vi "ReadArray.vi"(1 "reference":refnum<vi>) -> (0 "Array":T6)   [LabVIEW 2013]
uses:
  <vilib>/Utility/miscctls.llb/LVBoundsTypeDef.ctl
  <vilib>/Utility/miscctls.llb/LVPositionTypeDef.ctl
  <vilib>/Utility/miscctls.llb/LVRectTypeDef.ctl
  <vilib>/Utility/miscctls.llb/LVDataSocketStatusTypeDef.ctl
  <vilib>/Utility/miscctls.llb/LVKeyNavTypeDef.ctl
panel:
  out "error out 74":errorcluster
  out "error out 73":errorcluster
  out "error out 72":errorcluster
  out "error out 71":errorcluster
  out "error out 70":errorcluster
  out "error out 69":errorcluster
  out "error out 68":errorcluster
  out "error out 67":errorcluster
  out "error out 66":errorcluster
  out "error out 65":errorcluster
  out "error out 64":errorcluster
  out "error out 63":errorcluster
  out "error out 62":errorcluster
  out "error out 61":errorcluster
  out "error out 60":errorcluster
  out "error out 59":errorcluster
  out "error out 58":errorcluster
  out "error out 57":errorcluster
  out "error out 56":errorcluster
  out "error out 55":errorcluster
  out "error out 54":errorcluster
  out "error out 53":errorcluster
  out "error out 52":errorcluster
  out "error out 51":errorcluster
  out "error out 50":errorcluster
  out "error out 49":errorcluster
  out "error out 48":errorcluster
  out "error out 47":errorcluster
  out "error out 46":errorcluster
  out "error out 45":errorcluster
  out "error out 44":errorcluster
  out "error out 43":errorcluster
  out "error out 42":errorcluster
  out "error out 41":errorcluster
  out "error out 40":errorcluster
  out "error out 39":errorcluster
  out "error out 38":errorcluster
  out "error out 37":errorcluster
  out "error out 36":errorcluster
  out "error out 35":errorcluster
  out "error out 34":errorcluster
  out "error out 33":errorcluster
  out "error out 32":errorcluster
  out "error out 31":errorcluster
  out "error out 30":errorcluster
  out "error out 29":errorcluster
  out "error out 28":errorcluster
  out "error out 27":errorcluster
  out "error out 26":errorcluster
  out "error out 25":errorcluster
  out "error out 24":errorcluster
  out "error out 23":errorcluster
  out "error out 22":errorcluster
  out "error out 21":errorcluster
  out "error out 20":errorcluster
  out "error out 19":errorcluster
  out "error out 18":errorcluster
  out "error out 17":errorcluster
  out "error out 16":errorcluster
  out "error out 15":errorcluster
  out "error out 14":errorcluster
  out "error out 13":errorcluster
  out "error out 12":errorcluster
  out "error out 11":errorcluster
  out "error out 10":errorcluster
  out "error out 9":errorcluster
  out "error out 8":errorcluster
  out "error out 7":errorcluster
  out "error out 6":errorcluster
  out "error out 5":errorcluster
  out "error out 4":errorcluster
  out "error out 3":errorcluster
  out "error out 2":errorcluster
  out "error out":errorcluster
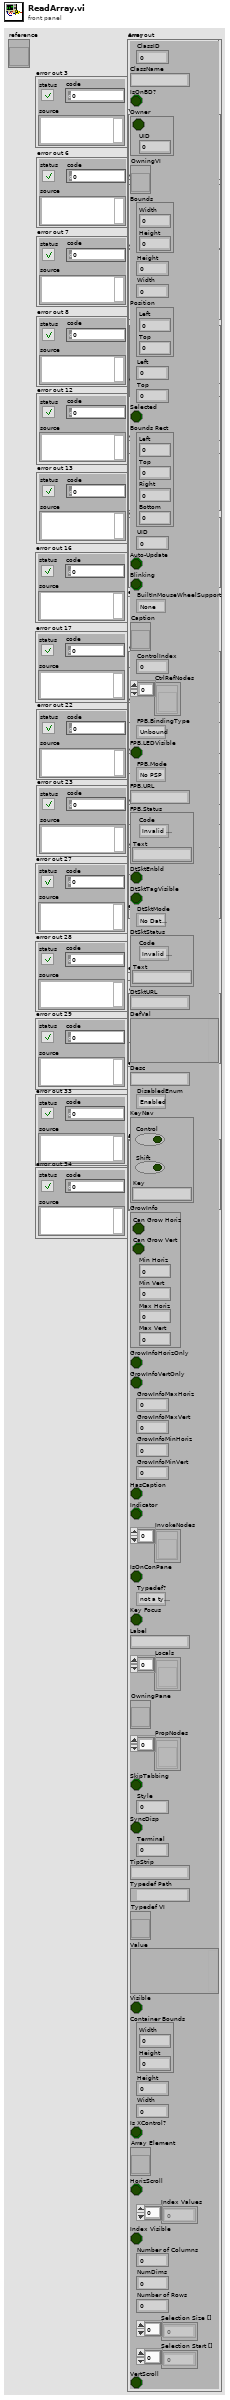
[diagram p1: front panel]
types:
  T1 = typedef "LVBoundsTypeDef.ctl" = cluster{"Width":u32, "Height":u32}
  T2 = typedef "LVPositionTypeDef.ctl" = cluster{"Left":i32, "Top":i32}
  T3 = typedef "LVRectTypeDef.ctl" = cluster{"Left":i16, "Top":i16, "Right":i16, "Bottom":i16}
  T4 = typedef "LVDataSocketStatusTypeDef.ctl" = cluster{"Code":enum32{"Invalid Status", "Unconnected", "Active", "Idle", "Error", "Connecting"}, "Text":string}
  T5 = typedef "LVKeyNavTypeDef.ctl" = cluster{"Control":bool, "Shift":bool, "Key":string}
  T6 = cluster{"ClassID":u32, "ClassName":string, "IsOnBD?":bool, "Owner":cluster{bool, "UID":i32}, "OwningVI":refnum<vi>, "Bounds":T1, "Height":u32, "Width":u32, "Position":T2, "Left":i32, "Top":i32, "Selected":bool, "Bounds Rect":T3, "UID":i32, "Auto-Update":bool, "Blinking":bool, "BuiltInMouseWheelSupport":enum16{"None", "On Hover", "On Key Focus", "On Hover or Key Focus"}, "Caption":refnum<vi>, "ControlIndex":i32, "CtrlRefNodes":refnum<vi>[], "FPB.BindingType":enum32{"Unbound", "Bound To PSP URL", "Bound To Variable Shortcut"}, "FPB.LEDVisible":bool, "FPB.Mode":enum32{"No PSP", "Read", "Write", "Write & Read"}, "FPB.URL":string, "FPB.Status":T4, "DtSktEnbld":bool, "DtSktTagVisible":bool, "DtSktMode":enum32{"No DataSocket", "Publish", "Subscribe", "Publish & Subscribe"}, "DtSktStatus":T4, "DtSktURL":string, "DefVal":variant, "Desc":string, "DisabledEnum":enum8{"Enabled", "Disabled", "Disabled and Grayed Out"}, "KeyNav":T5, "GrowInfo":cluster{"Can Grow Horiz":bool, "Can Grow Vert":bool, "Min Horiz":i16, "Min Vert":i16, "Max Horiz":i16, "Max Vert":i16}, "GrowInfoHorizOnly":bool, "GrowInfoVertOnly":bool, "GrowInfoMaxHoriz":i16, "GrowInfoMaxVert":i16, "GrowInfoMinHoriz":i16, "GrowInfoMinVert":i16, "HasCaption":bool, "Indicator":bool, "InvokeNodes":refnum<vi>[], "IsOnConPane":bool, "Typedef?":enum32{"not a typedef", "typedef", "strict typedef", "class private data"}, "Key Focus":bool, "Label":string, "Locals":refnum<vi>[], "OwningPane":refnum<vi>, "PropNodes":refnum<vi>[], "SkipTabbing":bool, "Style":u32, "SyncDisp":bool, "Terminal":i32, "TipStrip":string, "Typedef Path":path, "Typedef VI":refnum<vi>, "Value":variant, "Visible":bool, "Container Bounds":T1, "Height":u32, "Width":u32, "Is XControl?":bool, "Array Element":refnum<vi>, "HorizScroll":bool, "Index Values":u32[], "Index Visible":bool, "Number of Columns":u32, "NumDims":u32, "Number of Rows":u32, "Selection Size []":u32[], "Selection Start []":u32[], "VertScroll":bool}
  T7 = enum16{"None", "On Hover", "On Key Focus", "On Hover or Key Focus"}
  T8 = enum32{"No PSP", "Read", "Write", "Write & Read"}
  T9 = enum32{"Unbound", "Bound To PSP URL", "Bound To Variable Shortcut"}
  T10 = enum32{"No DataSocket", "Publish", "Subscribe", "Publish & Subscribe"}
  T11 = enum8{"Enabled", "Disabled", "Disabled and Grayed Out"}
  T12 = enum32{"not a typedef", "typedef", "strict typedef", "class private data"}
  T13 = cluster{"Can Grow Horiz":bool, "Can Grow Vert":bool, "Min Horiz":i16, "Min Vert":i16, "Max Horiz":i16, "Max Vert":i16}
  T14 = cluster{"ClassID":u32, "ClassName":string, "IsOnBD?":bool, "Cluster":cluster{bool, "UID":i32}, "OwningVI":refnum<vi>, "Bounds":T1, "Height":u32, "Width":u32, "Position":T2, "Left":i32, "Top":i32, "Selected":bool, "Bounds Rect":T3, "UID":i32, "Auto-Update":bool, "Blinking":bool, "BuiltInMouseWheelSupport":enum16{"None", "On Hover", "On Key Focus", "On Hover or Key Focus"}, "Caption":refnum<vi>, "ControlIndex":i32, "CtrlRefNodes":refnum<vi>[], "FPB.BindingType":enum32{"Unbound", "Bound To PSP URL", "Bound To Variable Shortcut"}, "FPB.LEDVisible":bool, "FPB.Mode":enum32{"No PSP", "Read", "Write", "Write & Read"}, "FPB.URL":string, "FPB.Status":T4, "DtSktEnbld":bool, "DtSktTagVisible":bool, "DtSktMode":enum32{"No DataSocket", "Publish", "Subscribe", "Publish & Subscribe"}, "DtSktStatus":T4, "DtSktURL":string, "DefVal":variant, "Desc":string, "DisabledEnum":enum8{"Enabled", "Disabled", "Disabled and Grayed Out"}, "KeyNav":T5, "GrowInfo":cluster{"Can Grow Horiz":bool, "Can Grow Vert":bool, "Min Horiz":i16, "Min Vert":i16, "Max Horiz":i16, "Max Vert":i16}, "GrowInfoHorizOnly":bool, "GrowInfoVertOnly":bool, "GrowInfoMaxHoriz":i16, "GrowInfoMaxVert":i16, "GrowInfoMinHoriz":i16, "GrowInfoMinVert":i16, "HasCaption":bool, "Indicator":bool, "InvokeNodes":refnum<vi>[], "IsOnConPane":bool, "Typedef?":enum32{"not a typedef", "typedef", "strict typedef", "class private data"}, "Key Focus":bool, "Text":string, "Locals":refnum<vi>[], "OwningPane":refnum<vi>, "PropNodes":refnum<vi>[], "SkipTabbing":bool, "Style":u32, "SyncDisp":bool, "UID":i32, "TipStrip":string, "Typedef Path":path, "Typedef VI":refnum<vi>, "Value":variant, "Visible":bool, "Container Bounds":T1, "Height":u32, "Width":u32, "Is XControl?":bool, "Array Element":refnum<vi>, "HorizScroll":bool, "Index Values":u32[], "Index Visible":bool, "Number of Columns":u32, "NumDims":u32, "Number of Rows":u32, "Selection Size []":u32[], "Selection Start []":u32[], "VertScroll":bool}
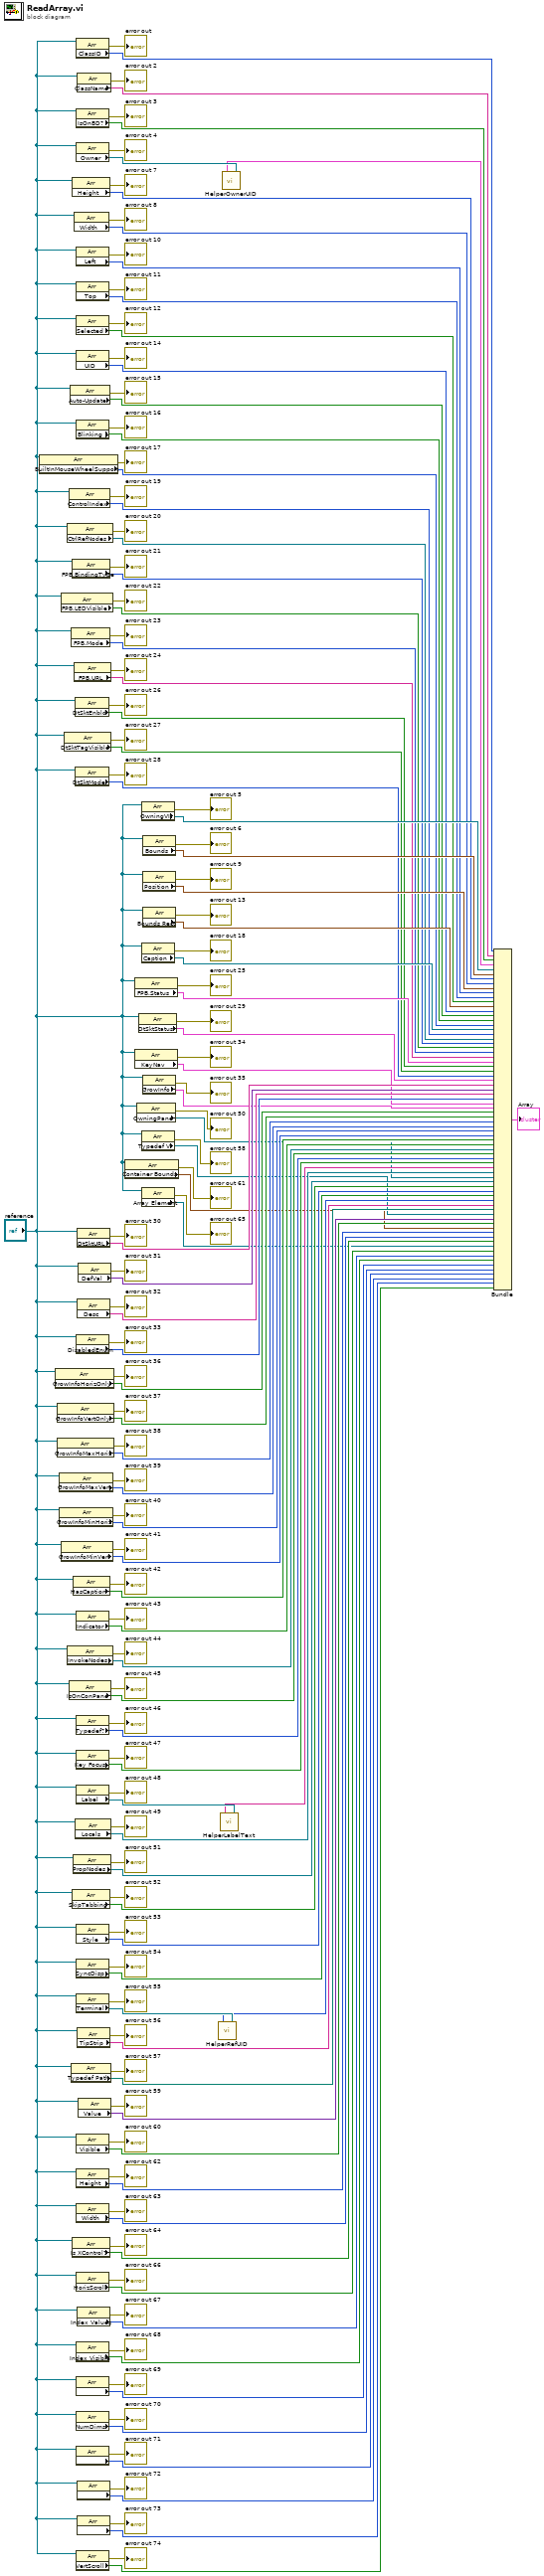
[diagram p0: block diagram]
diagram:
  n1 = property class="Arr"(reference="reference") -> (error out=→"error out 17":errorcluster, "BuiltInMouseWheelSupport"=w118:T7)  [unwired: 1 in, 1 out]
  n2 = property class="Arr"(reference="reference") -> (error out=→"error out 36":errorcluster, "GrowInfoHorizOnly"=w80:bool)  [unwired: 1 in, 1 out]
  n3 = property class="Arr"(reference="reference") -> (error out=→"error out 37":errorcluster, "GrowInfoVertOnly"=w78:bool)  [unwired: 1 in, 1 out]
  n4 = property class="Arr"(reference="reference") -> (error out=→"error out 38":errorcluster, "GrowInfoMaxHoriz"=w76:i16)  [unwired: 1 in, 1 out]
  n5 = property class="Arr"(reference="reference") -> (error out=→"error out 39":errorcluster, "GrowInfoMaxVert"=w74:i16)  [unwired: 1 in, 1 out]
  n6 = property class="Arr"(reference="reference") -> (error out=→"error out 40":errorcluster, "GrowInfoMinHoriz"=w72:i16)  [unwired: 1 in, 1 out]
  n7 = property class="Arr"(reference="reference") -> (error out=→"error out 22":errorcluster, "FPB.LEDVisible"=w108:bool)  [unwired: 1 in, 1 out]
  n8 = property class="Arr"(reference="reference") -> (error out=→"error out 41":errorcluster, "GrowInfoMinVert"=w70:i16)  [unwired: 1 in, 1 out]
  n9 = property class="Arr"(reference="reference") -> (error out=→"error out 27":errorcluster, "DtSktTagVisible"=w98:bool)  [unwired: 1 in, 1 out]
  n10 = property class="Arr"(reference="reference") -> (error out=→"error out 20":errorcluster, "CtrlRefNodes"=w112:refnum<vi>[])  [unwired: 1 in, 1 out]
  n11 = property class="Arr"(reference="reference") -> (error out=→"error out 44":errorcluster, "InvokeNodes"=w64:refnum<vi>[])  [unwired: 1 in, 1 out]
  n12 = property class="Arr"(reference="reference") -> (error out=→"error out 45":errorcluster, "IsOnConPane"=w62:bool)  [unwired: 1 in, 1 out]
  n13 = property class="Arr"(reference="reference") -> (error out=→"error out 19":errorcluster, "ControlIndex"=w114:i32)  [unwired: 1 in, 1 out]
  n14 = property class="Arr"(reference="reference") -> (error out=→"error out 15":errorcluster, "Auto-Update"=w122:bool)  [unwired: 1 in, 1 out]
  n15 = property class="Arr"(reference="reference") -> (error out=→"error out 23":errorcluster, "FPB.Mode"=w106:T8)  [unwired: 1 in, 1 out]
  n16 = property class="Arr"(reference="reference") -> (error out=→"error out 57":errorcluster, "Typedef Path"=w36:path)  [unwired: 1 in, 1 out]
  n17 = property class="Arr"(reference="reference") -> (error out=→"error out 7":errorcluster, "Height"=w138:u32)  [unwired: 1 in, 1 out]
  n18 = property class="Arr"(reference="reference") -> (error out=→"error out 21":errorcluster, "FPB.BindingType"=w110:T9)  [unwired: 1 in, 1 out]
  n19 = property class="Arr"(reference="reference") -> (error out=→"error out 52":errorcluster, "SkipTabbing"=w47:bool)  [unwired: 1 in, 1 out]
  n20 = property class="Arr"(reference="reference") -> (error out=→"error out 64":errorcluster, "Is XControl?"=w22:bool)  [unwired: 1 in, 1 out]
  n21 = property class="Arr"(reference="reference") -> (error out=→"error out 51":errorcluster, "PropNodes"=w49:refnum<vi>[])  [unwired: 1 in, 1 out]
  n22 = property class="Arr"(reference="reference") -> (error out=→"error out 42":errorcluster, "HasCaption"=w68:bool)  [unwired: 1 in, 1 out]
  n23 = property class="Arr"(reference="reference") -> (error out=→"error out 8":errorcluster, "Width"=w136:u32)  [unwired: 1 in, 1 out]
  n24 = property class="Arr"(reference="reference") -> (error out=→"error out 24":errorcluster, "FPB.URL"=w104:string)  [unwired: 1 in, 1 out]
  n25 = property class="Arr"(reference="reference") -> (error out=→"error out 26":errorcluster, "DtSktEnbld"=w100:bool)  [unwired: 1 in, 1 out]
  n26 = property class="Arr"(reference="reference") -> (error out=→"error out 28":errorcluster, "DtSktMode"=w96:T10)  [unwired: 1 in, 1 out]
  n27 = property class="Arr"(reference="reference") -> (error out=→"error out 49":errorcluster, "Locals"=w53:refnum<vi>[])  [unwired: 1 in, 1 out]
  n28 = property class="Arr"(reference="reference") -> (error out=→"error out":errorcluster, "ClassID"=w151:u32)  [unwired: 1 in, 1 out]
  n29 = property class="Arr"(reference="reference") -> (error out=→"error out 3":errorcluster, "IsOnBD?"=w147:bool)  [unwired: 1 in, 1 out]
  n30 = property class="Arr"(reference="reference") -> (error out=→"error out 4":errorcluster, "Owner"=w145:refnum<vi>)  [unwired: 1 in, 1 out]
  n31 = property class="Arr"(reference="reference") -> (error out=→"error out 10":errorcluster, "Left"=w132:i32)  [unwired: 1 in, 1 out]
  n32 = property class="Arr"(reference="reference") -> (error out=→"error out 11":errorcluster, "Top"=w130:i32)  [unwired: 1 in, 1 out]
  n33 = property class="Arr"(reference="reference") -> (error out=→"error out 12":errorcluster, "Selected"=w128:bool)  [unwired: 1 in, 1 out]
  n34 = property class="Arr"(reference="reference") -> (error out=→"error out 14":errorcluster, "UID"=w124:i32)  [unwired: 1 in, 1 out]
  n35 = property class="Arr"(reference="reference") -> (error out=→"error out 16":errorcluster, "Blinking"=w120:bool)  [unwired: 1 in, 1 out]
  n36 = property class="Arr"(reference="reference") -> (error out=→"error out 33":errorcluster, "DisabledEnum"=w86:T11)  [unwired: 1 in, 1 out]
  n37 = property class="Arr"(reference="reference") -> (error out=→"error out 43":errorcluster, "Indicator"=w66:bool)  [unwired: 1 in, 1 out]
  n38 = property class="Arr"(reference="reference") -> (error out=→"error out 46":errorcluster, "Typedef?"=w60:T12)  [unwired: 1 in, 1 out]
  n39 = property class="Arr"(reference="reference") -> (error out=→"error out 47":errorcluster, "Key Focus"=w58:bool)  [unwired: 1 in, 1 out]
  n40 = property class="Arr"(reference="reference") -> (error out=→"error out 48":errorcluster, "Label"=w56:refnum<vi>)  [unwired: 1 in, 1 out]
  n41 = property class="Arr"(reference="reference") -> (error out=→"error out 53":errorcluster, "Style"=w45:u32)  [unwired: 1 in, 1 out]
  n42 = property class="Arr"(reference="reference") -> (error out=→"error out 54":errorcluster, "SyncDisp"=w43:bool)  [unwired: 1 in, 1 out]
  n43 = property class="Arr"(reference="reference") -> (error out=→"error out 55":errorcluster, "Terminal"=w41:refnum<vi>)  [unwired: 1 in, 1 out]
  n44 = property class="Arr"(reference="reference") -> (error out=→"error out 60":errorcluster, "Visible"=w30:bool)  [unwired: 1 in, 1 out]
  n45 = property class="Arr"(reference="reference") -> (error out=→"error out 62":errorcluster, "Height"=w26:u32)  [unwired: 1 in, 1 out]
  n46 = property class="Arr"(reference="reference") -> (error out=→"error out 63":errorcluster, "Width"=w24:u32)  [unwired: 1 in, 1 out]
  n47 = property class="Arr"(reference="reference") -> (error out=→"error out 66":errorcluster, "HorizScroll"=w18:bool)  [unwired: 1 in, 1 out]
  n48 = property class="Arr"(reference="reference") -> (error out=→"error out 68":errorcluster, "Index Visible"=w14:bool)  [unwired: 1 in, 1 out]
  n49 = property class="Arr"(reference="reference") -> (error out=→"error out 69":errorcluster, "Number of Columns"=w12:u32)  [unwired: 1 in, 1 out]
  n50 = property class="Arr"(reference="reference") -> (error out=→"error out 70":errorcluster, "NumDims"=w10:u32)  [unwired: 1 in, 1 out]
  n51 = property class="Arr"(reference="reference") -> (error out=→"error out 71":errorcluster, "Number of Rows"=w8:u32)  [unwired: 1 in, 1 out]
  n52 = property class="Arr"(reference="reference") -> (error out=→"error out 74":errorcluster, "VertScroll"=w2:bool)  [unwired: 1 in, 1 out]
  n53 = property class="Arr"(reference="reference") -> (error out=→"error out 2":errorcluster, "ClassName"=w149:string)  [unwired: 1 in, 1 out]
  n54 = property class="Arr"(reference="reference") -> (error out=→"error out 30":errorcluster, "DtSktURL"=w92:string)  [unwired: 1 in, 1 out]
  n55 = property class="Arr"(reference="reference") -> (error out=→"error out 32":errorcluster, "Desc"=w88:string)  [unwired: 1 in, 1 out]
  n56 = property class="Arr"(reference="reference") -> (error out=→"error out 56":errorcluster, "TipStrip"=w38:string)  [unwired: 1 in, 1 out]
  n57 = property class="Arr"(reference="reference") -> (error out=→"error out 67":errorcluster, "Index Values"=w16:u32[])  [unwired: 1 in, 1 out]
  n58 = property class="Arr"(reference="reference") -> (error out=→"error out 72":errorcluster, "Selection Size []"=w6:u32[])  [unwired: 1 in, 1 out]
  n59 = property class="Arr"(reference="reference") -> (error out=→"error out 73":errorcluster, "Selection Start []"=w4:u32[])  [unwired: 1 in, 1 out]
  n60 = property class="Arr"(reference="reference") -> (error out=→"error out 31":errorcluster, "DefVal"=w90:variant)  [unwired: 1 in, 1 out]
  n61 = property class="Arr"(reference="reference") -> (error out=→"error out 59":errorcluster, "Value"=w32:variant)  [unwired: 1 in, 1 out]
  n62 = property class="Arr"(reference="reference") -> (error out=→"error out 61":errorcluster, "Container Bounds"=w28:T1)  [unwired: 1 in, 1 out]
  n63 = property class="Arr"(reference="reference") -> (error out=→"error out 25":errorcluster, "FPB.Status"=w102:T4)  [unwired: 1 in, 1 out]
  n64 = property class="Arr"(reference="reference") -> (error out=→"error out 34":errorcluster, "KeyNav"=w84:T5)  [unwired: 1 in, 1 out]
  n65 = property class="Arr"(reference="reference") -> (error out=→"error out 50":errorcluster, "OwningPane"=w51:refnum<vi>)  [unwired: 1 in, 1 out]
  n66 = property class="Arr"(reference="reference") -> (error out=→"error out 29":errorcluster, "DtSktStatus"=w94:T4)  [unwired: 1 in, 1 out]
  n67 = property class="Arr"(reference="reference") -> (error out=→"error out 5":errorcluster, "OwningVI"=w142:refnum<vi>)  [unwired: 1 in, 1 out]
  n68 = property class="Arr"(reference="reference") -> (error out=→"error out 18":errorcluster, "Caption"=w116:refnum<vi>)  [unwired: 1 in, 1 out]
  n69 = property class="Arr"(reference="reference") -> (error out=→"error out 58":errorcluster, "Typedef VI"=w34:refnum<vi>)  [unwired: 1 in, 1 out]
  n70 = property class="Arr"(reference="reference") -> (error out=→"error out 65":errorcluster, "Array Element"=w20:refnum<vi>)  [unwired: 1 in, 1 out]
  n71 = property class="Arr"(reference="reference") -> (error out=→"error out 6":errorcluster, "Bounds"=w140:T1)  [unwired: 1 in, 1 out]
  n72 = property class="Arr"(reference="reference") -> (error out=→"error out 9":errorcluster, "Position"=w134:T2)  [unwired: 1 in, 1 out]
  n73 = property class="Arr"(reference="reference") -> (error out=→"error out 13":errorcluster, "Bounds Rect"=w126:T3)  [unwired: 1 in, 1 out]
  n74 = property class="Arr"(reference="reference") -> (error out=→"error out 35":errorcluster, "GrowInfo"=w82:T13)  [unwired: 1 in, 1 out]
  n75 = call "HelperRefUID.vi"("Text in"=w41) -> ("UID"=w40:i32)
  n76 = call "HelperLabelText.vi"("Text in"=w56) -> ("Text"=w55:string)
  n77 = call "HelperOwnerUID.vi"("Generic in"=w145) -> ("Cluster"=w144:cluster{bool, "UID":i32})
  n78 = Bundle("ClassID"=w151, "ClassName"=w149, "IsOnBD?"=w147, "Cluster"=w144, "OwningVI"=w142, "Bounds"=w140, "Height"=w138, "Width"=w136, "Position"=w134, "Left"=w132, "Top"=w130, "Selected"=w128, "Bounds Rect"=w126, "UID"=w124, "Auto-Update"=w122, "Blinking"=w120, "BuiltInMouseWheelSupport"=w118, "Caption"=w116, "ControlIndex"=w114, "CtrlRefNodes"=w112, "FPB.BindingType"=w110, "FPB.LEDVisible"=w108, "FPB.Mode"=w106, "FPB.URL"=w104, "FPB.Status"=w102, "DtSktEnbld"=w100, "DtSktTagVisible"=w98, "DtSktMode"=w96, "DtSktStatus"=w94, "DtSktURL"=w92, "DefVal"=w90, "Desc"=w88, "DisabledEnum"=w86, "KeyNav"=w84, "GrowInfo"=w82, "GrowInfoHorizOnly"=w80, "GrowInfoVertOnly"=w78, "GrowInfoMaxHoriz"=w76, "GrowInfoMaxVert"=w74, "GrowInfoMinHoriz"=w72, "GrowInfoMinVert"=w70, "HasCaption"=w68, "Indicator"=w66, "InvokeNodes"=w64, "IsOnConPane"=w62, "Typedef?"=w60, "Key Focus"=w58, "Text"=w55, "Locals"=w53, "OwningPane"=w51, "PropNodes"=w49, "SkipTabbing"=w47, "Style"=w45, "SyncDisp"=w43, "UID"=w40, "TipStrip"=w38, "Typedef Path"=w36, "Typedef VI"=w34, "Value"=w32, "Visible"=w30, "Container Bounds"=w28, "Height"=w26, "Width"=w24, "Is XControl?"=w22, "Array Element"=w20, "HorizScroll"=w18, "Index Values"=w16, "Index Visible"=w14, "Number of Columns"=w12, "NumDims"=w10, "Number of Rows"=w8, "Selection Size []"=w6, "Selection Start []"=w4, "VertScroll"=w2) -> (→"Array":T14)  [unwired: 1 in]
